vi "rgb2array.vi"(5 "Image IN":T1(plugin-control), 11 "error in (no error)":errorcluster) -> (6 "output Array":dbl[][][](array[numeric]), 15 "error out":errorcluster)   [LabVIEW 2019]
uses:
  <vilib>/vision/NI_Vision_Development_Module.lvlib
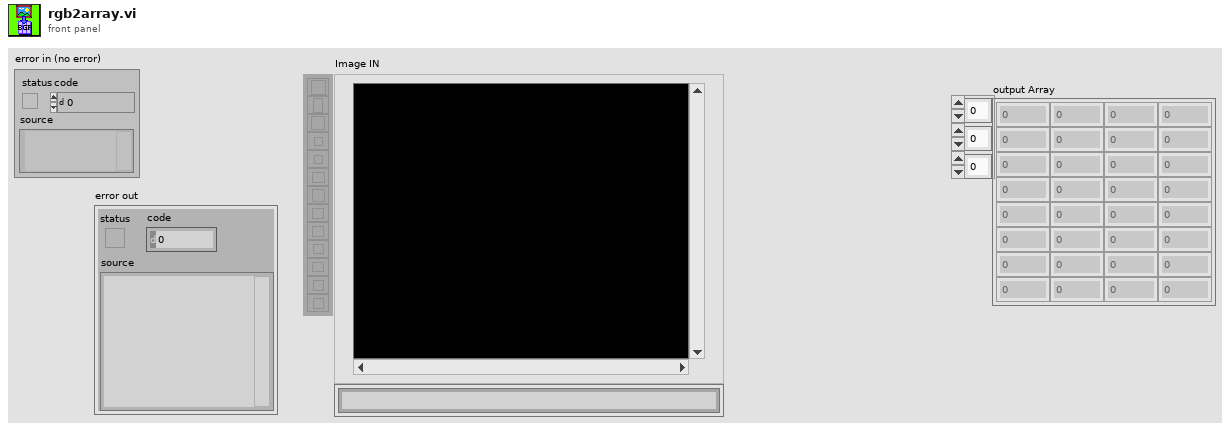
[diagram p1: front panel]
types:
  T1 = typedef "IMAQ Image.ctl" = refnum<image>
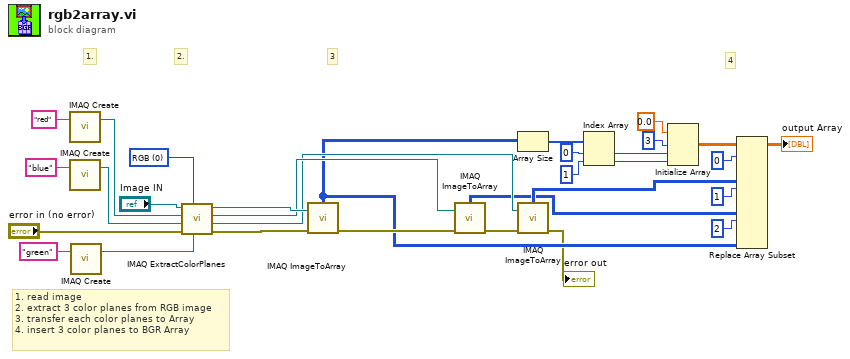
[diagram p0: block diagram]
diagram:
  w31 = u16 0 items=["RGB", "HSL", "HSV", "HSI"] ("Color Mode")
  # "1. read image\n2. extract 3 color planes from RGB image\n3. transfer each color planes to Array\n4. insert 3 color planes to BGR Array"
  # "4"
  # "3"
  # "2."
  # "1."
  n1 = call "IMAQ Create"("Image Name"="red") -> ("New Image"=w29:T1)  [unwired: 4 in, 1 out]
  n2 = call "IMAQ Create"("Image Name"="blue") -> ("New Image"=w26:T1)  [unwired: 4 in, 1 out]
  n3 = call "IMAQ Create"("Image Name"="green") -> ("New Image"=w25:T1)  [unwired: 4 in, 1 out]
  n4 = call "IMAQ ExtractColorPlanes"("Blue or Luma or Val or Inten Plane"=w25, "Color Mode"=w31, "error in (no error)"="error in (no error)", "Green or Sat Plane"=w26, "Red or Hue Plane"=w29, "Image Src"="Image IN") -> ("error out"=w23:errorcluster, "Blue or Luma or Val or Inten Plane out"=w19:T1, "Green or Sat Plane out"=w22:T1, "Red or Hue Plane out"=w24:T1)  [unwired: 2 in]
  n5 = call "IMAQ ImageToArray"("error in (no error)"=w23, "Image"=w24) -> ("error out"=w21:errorcluster, "Image Pixels (U8)"=w5:u8[][])  [unwired: 2 in, 3 out]
  n6 = call "IMAQ ImageToArray"("error in (no error)"=w21, "Image"=w22) -> ("error out"=w20:errorcluster, "Image Pixels (U8)"=w6:u8[][])  [unwired: 2 in, 3 out]
  n7 = Array Size(array=w5) -> (size(s)=w17:i32[])
  n8 = call "IMAQ ImageToArray"("error in (no error)"=w20, "Image"=w19) -> ("error out"=→"error out":errorcluster, "Image Pixels (U8)"=w10:u8[][])  [unwired: 2 in, 3 out]
  n9 = Index Array(array=w17, index #1=0 ("index"), index #2=1 ("index")) -> (element #1=w13:i32, element #2=w12:i32)
  n10 = Initialize Array(0.0 ("element"), 3 ("dimension size"), w13, w12) -> (w11:dbl[][][])
  n11 = Replace Array Subset(array=w11, new element #1=w10, index (dim 0) #1=0 ("index (page)"), new element #2=w6, index (dim 0) #2=1 ("index (page)"), new element #3=w5, index (dim 0) #3=2 ("index (page)")) -> (→"output Array":dbl[][][])  [unwired: 6 in]
